vi "脉冲生成_基于频率_单脉冲.vi"() -> ()   [LabVIEW 2013]
uses:
  <userlib>/ArtDAQ/_SubVI/ArtDAQ_CreateCOPulseChanFreq.vi
  <userlib>/ArtDAQ/_SubVI/ArtDAQ_CfgDigEdgeStartTrig.vi
panel:
  in  "触发模式":enum32{"No Trigger", "DigStartTrig"}(tab)=enum."DigStartTrig"
  in  "触发边沿":i32(ring)=10280 items=["上升"=10280, "下降"=10171]
  in  "触发源":string(combo)="/Dev1/PFI1"
  in  "可重?":bool
  in  "Stop":bool
  in  "计数器":string="Dev1/ctr0"
  in  "占空比":dbl=0.5 format="%0.6f"
  in  "频率":dbl=100.0 format="%0.6f"
  out "错误输出":errorcluster
  # "通道属性"
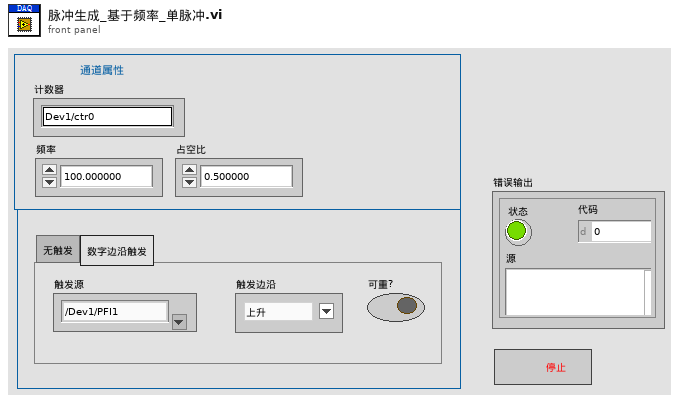
[diagram p1: front panel]
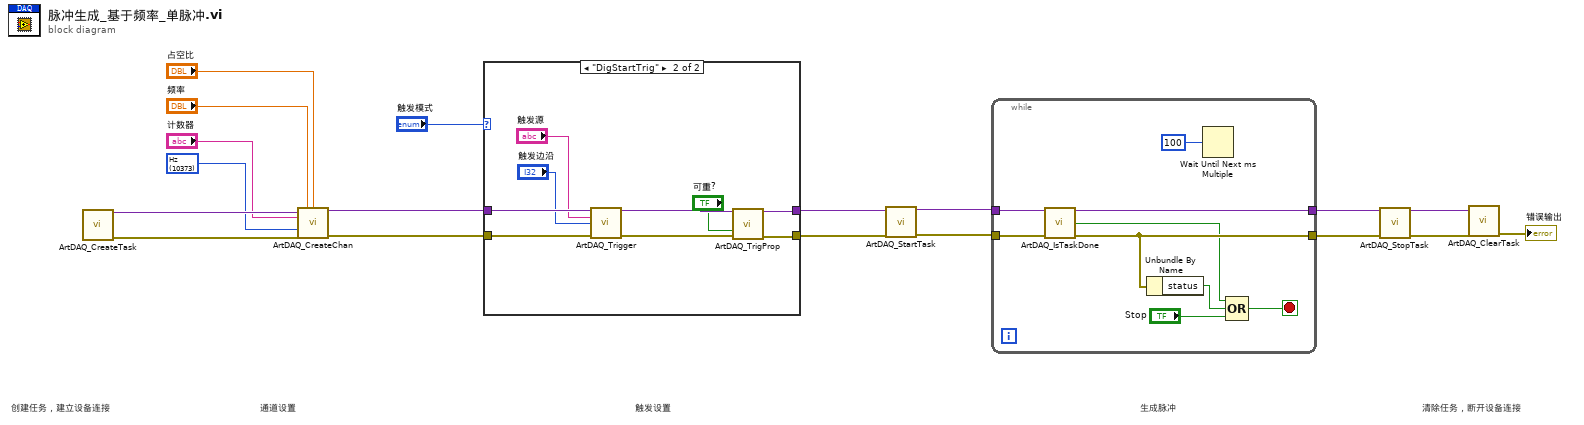
[diagram p0: block diagram]
diagram:
  w8 = 10373 items=["Hz"=10373] ("Units")
  # "清除任务，断开设备连接"
  # "生成脉冲"
  # "触发设置"
  # "通道设置"
  # "创建任务，建立设备连接"
  n1 = call <userlib>:"ArtDAQ_CreateTask.vi"() -> ("任务句柄"=w18:variant, "错误输出"=w17:errorcluster)  [unwired: 14 in]
  n2 = call-poly <userlib>:"ArtDAQ_CreateChan.vi"("任务句柄"=w18, "频率"="频率", "占空比"="占空比", "计数器"="计数器", "单位"=w8, "错误输入"=w17) -> ("任务句柄"=w6:variant, "错误输出"=w5:errorcluster)  [unwired: 8 in]
  n3 = case shown="\"DigStartTrig\"" "触发模式" {
    tunnel: w6 -> [w20 w29]
    tunnel: [w20 w22] -> w4
    tunnel: [w19 w24] -> w1
    tunnel: w5 -> [w19 w28]
    frame "No Trigger", Default {
    }
    frame "DigStartTrig" {
      n4 = call-poly <userlib>:"ArtDAQ_Trigger.vi"("任务句柄"=w29, "触发源"="触发源", "边沿"="触发边沿", "错误输入"=w28) -> ("任务句柄"=w23:variant, "错误输出"=w25:errorcluster)  [unwired: 10 in]
      n5 = call-poly <userlib>:"ArtDAQ_TrigProp.vi"("任务句柄"=w23, "可重?"="可重?", "错误输入"=w25) -> ("任务句柄"=w22:variant, "错误输出"=w24:errorcluster)  [unwired: 11 in]
    }
  }
  n6 = call <userlib>:"ArtDAQ_StartTask.vi"("任务句柄"=w4, "错误输入"=w1) -> ("任务句柄"=w3:variant, "错误输出"=w2:errorcluster)  [unwired: 12 in]
  n7 = while {
    tunnel: [w38] -> w15
    tunnel: [w37] -> w13
    tunnel: w3 -> [w34]
    tunnel: w2 -> [w33]
    stop <- w32 stop-if-true
    n8 = call <userlib>:"ArtDAQ_IsTaskDone.vi"("任务句柄"=w34, "错误输入"=w33) -> ("任务句柄"=w38:variant, "完成任务？"=w30:bool, "错误输出"=w37:errorcluster)  [unwired: 11 in]
    n9 = Unbundle By Name(w37) -> ("status"=w36:bool)
    n10 = Wait Until Next ms Multiple(millisecond multiple=u32 100 ("毫秒倍数")) -> ()  [unwired: 1 out]
    n11 = Compound Arithmetic op=OR(w30, w36, "Stop") -> (w32:bool)
  }
  n12 = call <userlib>:"ArtDAQ_StopTask.vi"("任务句柄"=w15, "错误输入"=w13) -> ("任务句柄"=w14:variant, "错误输出"=w12:errorcluster)  [unwired: 12 in]
  n13 = call <userlib>:"ArtDAQ_ClearTask.vi"("任务句柄"=w14, "错误输入"=w12) -> ("错误输出"=→"错误输出":errorcluster)  [unwired: 13 in]
